vi "test Parse Sorted Object Dictionary_4.vi"(11 "Test Case In":refnum<class "test EDS.lvclass">) -> (0 "error out":errorcluster, 3 "Test Case Out":refnum<class "test EDS.lvclass">)   [LabVIEW 2024, in "test EDS.lvclass"]
uses:
  test EDS.lvclass
  C:/Program Files/National Instruments/LabVIEW 2024/vi.lib/Astemes/LUnit/Test Case.lvclass
  Core/EDS/EDS.lvclass
  Core/Object Type.ctl
  Core/Data Type.ctl
  Core/Access Type.ctl
  Core/EDS/EDS.lvclass/EDS.ctl
  <vilib>/Astemes/LUnit/Test Case.lvclass/Test Case.ctl
  <vilib>/Astemes/LUnit/Append Fail Result.vi
  <vilib>/Astemes/LUnit/Append Pass Result.vi
  <vilib>/Astemes/LUnit/Run In UI.vi
  <vilib>/Utility/error.llb/Clear Errors.vi
  Core/OD Sub-Entry/OD Sub-Entry.lvclass
  D:/git/EDS-File-Viewer/Core/OD Entry/OD Entry.lvclass
  Core/OD Entry/Get PDOMapping.vi
  Core/OD Entry/Get DefaultValue.vi
  Core/OD Entry/Get AccessType.vi
  Core/OD Entry/Get DataType.vi
  Core/OD Entry/Get ObjectType.vi
  Core/OD Entry/Get ParameterName.vi
  <vilib>/Astemes/LUnit/Test Case.lvclass
  Core/EDS.lvlib
  Core/OD Entry/OD Entry.lvclass
  Core/Sorted Object Dictionary/Sorted Object Dictionary.lvclass
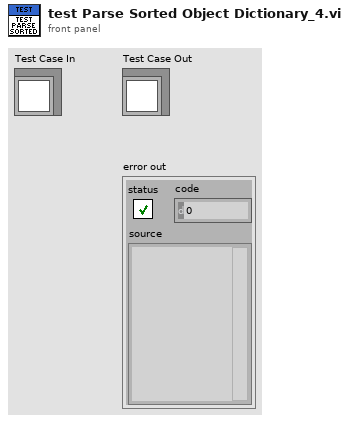
[diagram p1: front panel]
types:
  T1 = typedef "EDS.lvlib/Access Type.ctl" = enum16{"ro", "wo", "rw", "rwr", "rww", "const"}
  T2 = typedef "EDS.lvlib/Data Type.ctl" = u16
  T3 = typedef "EDS.lvlib/Object Type.ctl" = u8
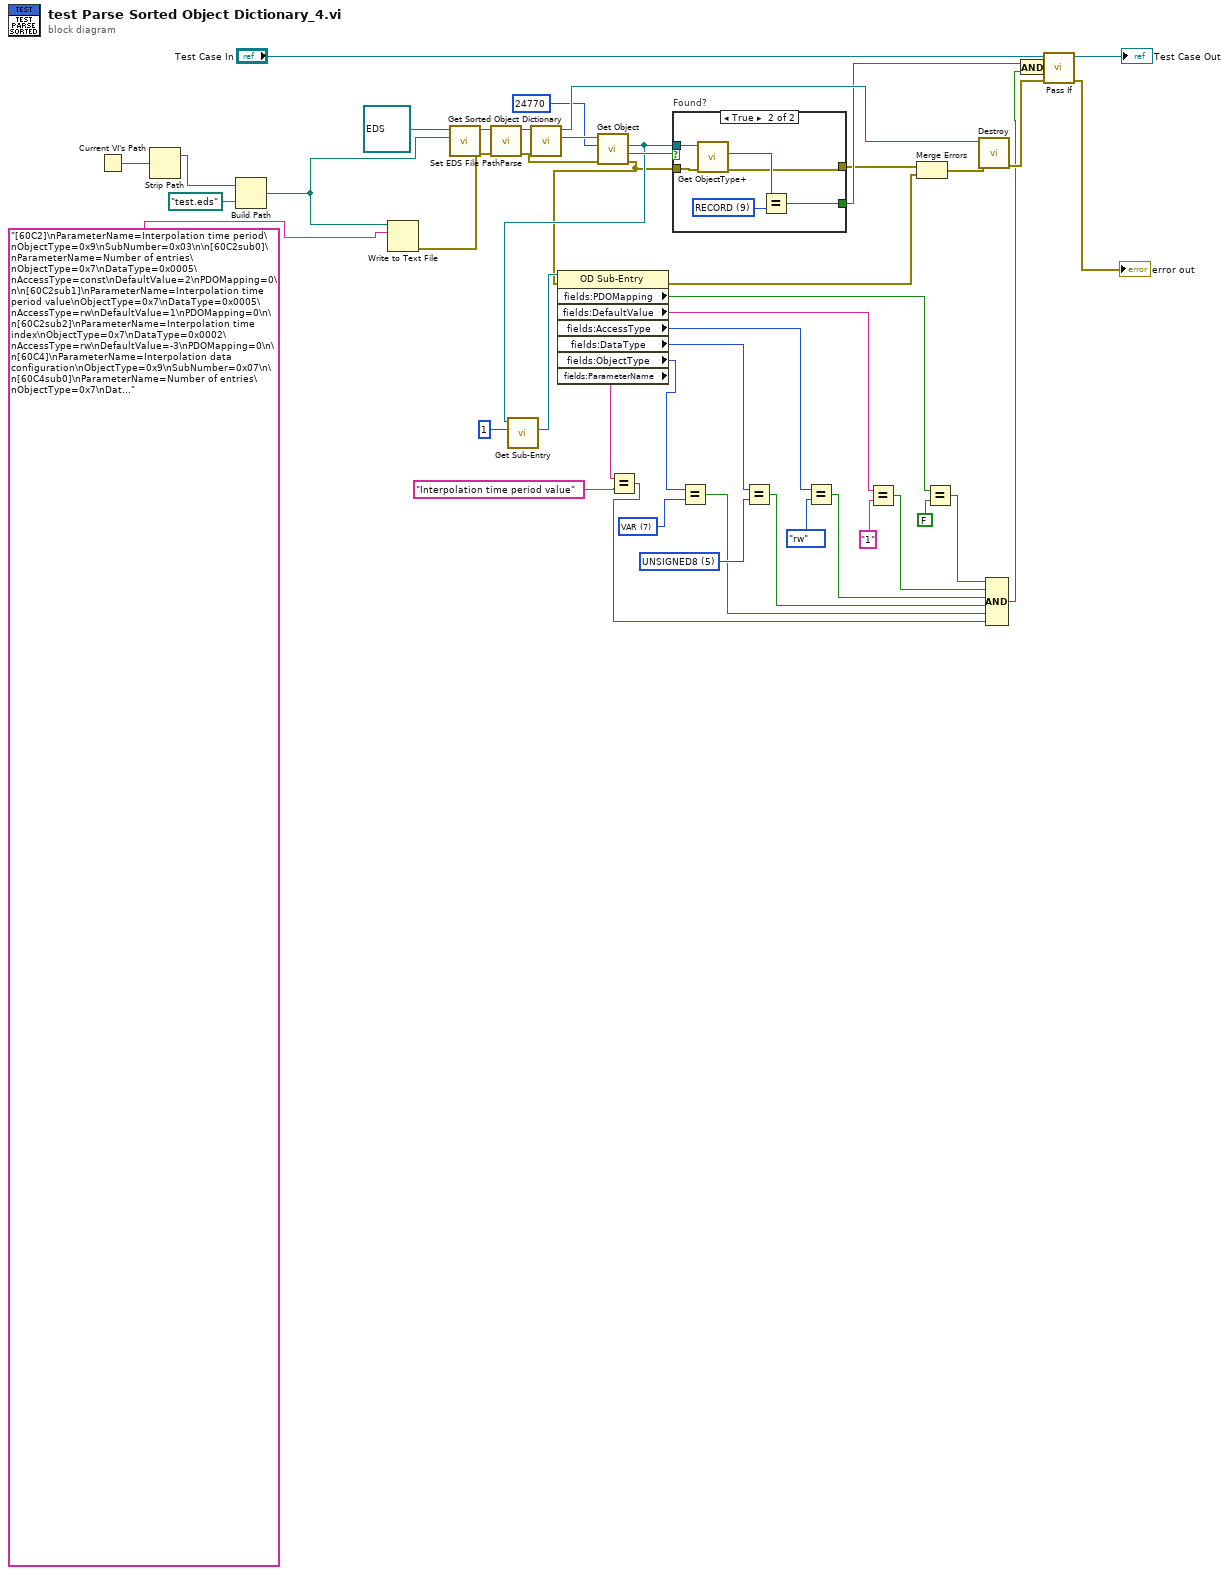
[diagram p0: block diagram]
diagram:
  w25 = T2 5 items=["BOOLEAN"=1, "INTEGER8"=2, "INTEGER16"=3, "INTEGER32"=4, "UNSIGNED8"=5, "UNSIGNED16"=6, "UNSIGNED32"=7, "REAL32"=8, "VISIBLE_STRING"=9, "OCTET_STRING"=10, "UNICODE_STRING"=11, "TIME_OF_DAY"=12, "TIME_DIFFERENCE"=13, "RESERVED1"=14, "DOMAIN"=15, "INTEGER24"=16, "REAL64"=17, "INTEGER40"=18, "INTEGER48"=19, "INTEGER56"=20, "INTEGER64"=21, "UNSIGNED24"=22, "RESERVED2"=23, "UNSIGNED40"=24, "UNSIGNED48"=25, "UNSIGNED56"=26, "UNSIGNED64"=27, "RESERVED3"=28, "RESERVED4"=29, "RESERVED5"=30, "RESERVED6"=31, "PDO_COMMUNICATION_PARAMETER"=32, "PDO_MAPPING"=33, "SDO_PARAMETER"=34, "IDENTITY"=35, "RESERVED7"=36] ("DataType")
  w26 = T3 7 items=["NULL"=0, "DOMAIN"=2, "DEFTYPE"=5, "DEFSTRUCT"=6, "VAR"=7, "ARRAY"=8, "RECORD"=9] ("ObjectType")
  n1 = Current VI's Path() -> (path=w41:path)
  n2 = Strip Path(path=w41) -> (stripped path=w37:path)  [unwired: 1 out]
  n3 = Build Path(base path=w37, name or relative path=path "test.eds") -> (appended path=w38:path)
  n4 = Write to Text File(file (use dialog)=w38, text="[60C2]\nParameterName=Interpolation time period\nObjectType=0x9\nSubNumber=0x03\n\n[60C2sub0]\nParameterName=Number of entries\nObjectType=0x7\nDataType=0x0005\nAccessType=const\nDefaultValue=2\nPDOMapping=0\n\n[60C2sub1]\nParameterName=Interpolation time period value\nObjectType=0x7\nDataType=0x0005\nAccessType=rw\nDefaultValue=1\nPDOMapping=0\n\n[60C2sub2]\nParameterName=Interpolation time index\nObjectType=0x7\nDataType=0x0002\nAccessType=rw\nDefaultValue=-3\nPDOMapping=0\n\n[60C4]\nParameterName=Interpolation data configuration\nObjectType=0x9\nSubNumber=0x07\n\n[60C4sub0]\nParameterName=Number of entries\nObjectType=0x7\nDataType=0x0005\nAccessType=const\nDefaultValue=6\nPDOMapping=0\n\n[60C4sub1]\nParameterName=MaximumBufferSize\nObjectType=0x7\nDataType=0x0007\nAccessType=ro\nDefaultValue=1\nPDOMapping=0\n\n[60C4sub2]\nParameterName=ActualBufferSize\nObjectType=0x7\nDataType=0x0007\nAccessType=rw\nDefaultValue=1\nPDOMapping=0\n\n[60C4sub3]\nParameterName=BufferOrganization\nObjectType=0x7\nDataType=0x0005\nAccessType=rw\nDefaultValue=0\nPDOMapping=0\n\n[60C4sub4]\nParameterName=BufferPosition\nObjectType=0x7\nDataType=0x0006\nAccessType=rw\nDefaultValue=1\nPDOMapping=0\n\n[60C4sub5]\nParameterName=SizeOfDataRecord\nObjectType=0x7\nDataType=0x0005\nAccessType=wo\nDefaultValue=4\nPDOMapping=0\n\n[60C4sub6]\nParameterName=BufferClear\nObjectType=0x7\nDataType=0x0005\nAccessType=wo\nDefaultValue=0\nPDOMapping=0") -> (error out=w39:errorcluster)  [unwired: 2 in, 2 out]
  n5 = call "Set EDS File Path.vi"("EDS File Path"=w38, "EDS in"=refnum<class "EDS.lvclass"> refnum ("EDS.lvlib:EDS.lvclass")) -> ("EDS out"=w42:refnum<class "EDS.lvclass">)  [unwired: 9 in]
  n6 = call "Parse.vi"("error in"=w39, "EDS in"=w42) -> ("error out"=w2:errorcluster, "EDS out"=w36:refnum<class "EDS.lvclass">)  [unwired: 8 in]
  n7 = call "Get Sorted Object Dictionary.vi"("EDS in"=w36) -> ("Sorted Object Dictionary"=w33:refnum<class "Sorted Object Dictionary.lvclass">, "EDS out"=w35:refnum<class "EDS.lvclass">)  [unwired: 9 in]
  n8 = call "Get Object.vi"("error in"=w2, "Index"=u16 24770 ("Numeric"), "Sorted Object Dictionary in"=w33) -> ("error out"=w1:errorcluster, "Found?"=w29:bool, "OD Entry"=w12:refnum<class "OD Entry.lvclass">)  [unwired: 5 in, 1 out]
  n9 = call "Get Sub-Entry.vi"("Sub-Index"=u16 1, "reference in"=w12) -> ("OD Sub-Entry"=w11:refnum<class "OD Sub-Entry.lvclass">)  [unwired: 6 in, 3 out]
  n10 = property class="OD Sub-Entry"(reference=w11, error in=w1) -> (error out=w9:errorcluster, "fields:PDOMapping"=w10:bool, "fields:DefaultValue"=w8:string, "fields:AccessType"=w7:T1, "fields:DataType"=w6:T2, "fields:ObjectType"=w5:T3, "fields:ParameterName"=w4:string)  [unwired: 1 out]
  n11 = Equal?(x=w4, y="Interpolation time period value") -> (x = y?=w20:bool)
  n12 = case "Found?" shown="True" w29 {
    selector: w29 -> [w47 _]
    tunnel: w12 -> [_ w54]
    tunnel: w1 -> [w48 w53]
    tunnel: [w47 w49] -> w32
    tunnel: [w48 w50] -> w30
    frame False {
    }
    frame True {
      w51 = T3 9 items=["NULL"=0, "DOMAIN"=2, "DEFTYPE"=5, "DEFSTRUCT"=6, "VAR"=7, "ARRAY"=8, "RECORD"=9] ("y")
      n13 = call "Get ObjectType+.vi"("Error In"=w53, "reference in"=w54) -> ("Error Out"=w50:errorcluster, "ObjectType"=w52:T3)  [unwired: 6 in, 2 out]
      n14 = Equal?(x=w52, y=w51) -> (x = y?=w49:bool)
    }
  }
  n15 = Equal?(x=w5, y=w26) -> (x = y?=w19:bool)
  n16 = Equal?(x=w6, y=w25) -> (x = y?=w18:bool)
  n17 = Equal?(x=w7, y=Access_Type."rw") -> (x = y?=w17:bool)
  n18 = Equal?(x=w8, y="1") -> (x = y?=w16:bool)
  n19 = Merge Errors(w30, w9) -> (w14:errorcluster)
  n20 = Equal?(x=w10, y=FALSE) -> (x = y?=w15:bool)
  n21 = call "Destroy.vi"("error in"=w14, "EDS in"=w35) -> ("error out"=w31:errorcluster)  [unwired: 8 in, 1 out]
  n22 = Compound Arithmetic op=AND(w15, w16, w17, w18, w19, w20) -> (w21:bool)
  n23 = And(x=w32, y=w21) -> (x .and. y?=w13:bool)
  n24 = call <vilib>:"Pass If.vi"("error in (no error)"=w31, "Pass?"=w13, "LUnit Test Case In"="Test Case In") -> ("error out"=→"error out":errorcluster, "LUnit Test Case Out"=→"Test Case Out":refnum<class "test EDS.lvclass">)  [unwired: 7 in]
